vi "savingArray(ofAnything)ToINIfile.vi"() -> ()   [LabVIEW 2021]
uses:
  <vilib>/Utility/config.llb/NI_LVConfig.lvlib
panel:
  out "Cluster":cluster{"Numeric":dbl, "String":string}
  in  "myArray":cluster{"Numeric":dbl, "String":string}[](array[cluster])=[{"Numeric"=0.0, "String"="zero"}, {"Numeric"=1.0, "String"="one"}, {"Numeric"=2.0, "String"="two"}]
  # "If you typedef your cluster, then this will look after itself at least... but is specific to that typedef, of course"
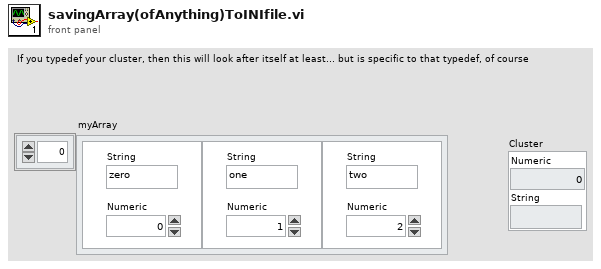
[diagram p1: front panel]
types:
  T1 = typedef "NI_LVConfig.lvlib/Config Data RefNum.ctl" = refnum<k1>
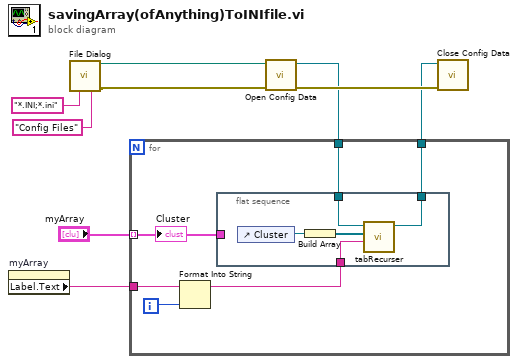
[diagram p0: block diagram]
diagram:
  n1 = property on="myArray" class="Arr (strict)"() -> ("Label.Text"=w8:string)  [unwired: 2 in, 2 out]
  n2 = call "File Dialog"("pattern (all files)"="*.INI;*.ini", "pattern label"="Config Files") -> ("selected path"=w2:path, "error out"=w1:errorcluster)  [unwired: 10 in, 2 out]
  n3 = call <vilib>:"Open Config Data.vi"("error in (no error)"=w1, "configuration file path"=w2) -> ("error out"=w7:errorcluster, "refnum"=w6:T1)  [unwired: 7 in, 1 out]
  n4 = for {
    tunnel: "myArray" -> [w12] mode=indexing
    tunnel: w8 -> [w15]
    tunnel: w6 -> [w11]
    tunnel: [w10] -> w5
    i -> [w14]
    n5 = Format Into String(initial string=w15, w14) -> (resulting string=w13:string)  [unwired: 2 in, 1 out]
    n6 = flat-sequence {
      tunnel: w13 -> [w18]
      tunnel: w12 -> [_]
      tunnel: w11 -> [w17]
      tunnel: [w16] -> w10
      frame #0 {
        n7 = control-ref of="Cluster"() -> (w20:refnum<vi>)
        n8 = Build Array(w20) -> (w19:refnum<vi>[])
        n9 = call "tabRecurser.vi"("SectionNameIn"=w18, "controlsIn[]"=w19, "INIrefnumIn"=w17) -> ("INIrefnumOut"=w16:T1)  [unwired: 7 in, 1 out]
      }
    }
    "Cluster" <- w12
  }
  n10 = call <vilib>:"Close Config Data.vi"("error in (no error)"=w7, "refnum"=w5) -> ()  [unwired: 8 in, 2 out]
